vi "GetExtensionInfo.vi"(8 "error in (no error)":errorcluster, 11 "GXML in":refnum<class "GXML.lvclass">) -> (0 "error out":errorcluster, 2 "Extension Info":T1, 3 "GXML out":refnum<class "GXML.lvclass">)   [LabVIEW 2020, in "File Formats.lvlib" / "GXML.lvclass"]
uses:
  GXML.lvclass
  Parent/Extension Info.ctl
  Parent/FileFormat.lvclass
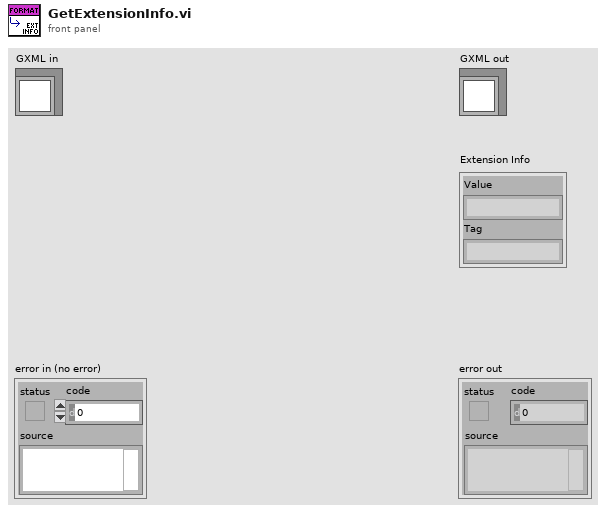
[diagram p1: front panel]
types:
  T1 = typedef "File Formats.lvlib/FileFormat.lvclass/Extension Info.ctl" = cluster{"Value":string, "Tag":string}
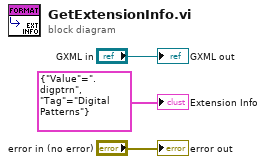
[diagram p0: block diagram]
diagram:
  "error out" <- "error in (no error)"
  "GXML out" <- "GXML in"
  "Extension Info" <- T1 {"Value"=".digptrn", "Tag"="Digital Patterns"} ("Extension Info")
